vi "Clear Tasks.vi"(8 "error in":errorcluster, 11 "PAS in":refnum<class "PAS.lvclass">) -> (0 "error out":errorcluster, 3 "PAS out":refnum<class "PAS.lvclass">)   [LabVIEW 2014, in "PAS.lvclass"]
doc: "If any signals used for housekeeping or high frequency acquisition (i.e. microphone or photodioded data) are captured using DAQmx, this will shut those tasks down properly."
uses:
  PAS.lvclass
  PAS.lvclass/PAS.ctl
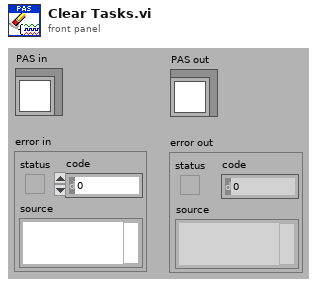
[diagram p1: front panel]
types:
  T1 = cluster{"acoustic":refnum<k21>, "housekeeping":refnum<k21>}
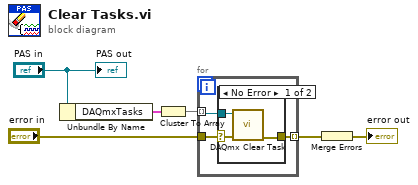
[diagram p0: block diagram]
diagram:
  n1 = Unbundle By Name("PAS in") -> ("DAQmxTasks"=w3:T1)
  n2 = Cluster To Array(cluster=w3) -> (array=w2:refnum<k21>[])
  n3 = for {
    tunnel: w2 -> [w7] mode=indexing
    tunnel: "error in" -> [w8]
    tunnel: [w9] -> w1 mode=indexing
    n4 = case shown="No Error" w8 {
      selector: w8 -> [w10 _]
      tunnel: [w12 _] -> w9
      tunnel: w7 -> [w11 _]
      frame No Error {
        n5 = call <vilib>:"DAQmx Clear Task.vi"("task in"=w11, "error in"=w10) -> ("error out"=w12:errorcluster)  [unwired: 13 in]
      }
      frame Error {
      }
    }
  }
  n6 = Merge Errors(w1) -> (→"error out":errorcluster)
  "PAS out" <- "PAS in"
